vi "InStuckInIronsMode.vi"(11 "RelativeWind (0-180)":dbl) -> (3 "InStuckInIronsMode?":bool)   [LabVIEW 2012]
doc: "Checks if the boat is 1) in irons and 2) is going very slowly. There are two cutoffs - an inner angle which has lower standards for what counts as 'in irons' and a broader angle with higher standards for what counts as 'in irons'. This way if the boat is going slowly but is around, say, 25 degrees off the wind, that won't count as stuck. That same speed at 8 degrees off the wind would count as stuck.\n\nIf the boat momentum is low and the boat is in irons range this algorithm should return TRUE and we should use the sails/rudder to coax ourselves out of irons.\n\nEric Schneider, Jan. 2014"
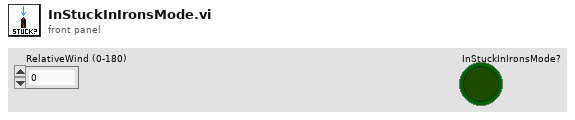
[diagram p1: front panel]
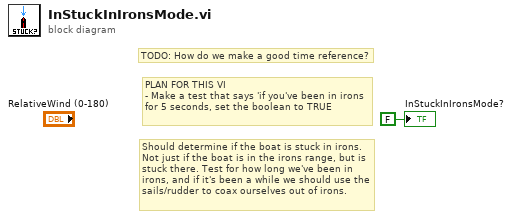
[diagram p0: block diagram]
diagram:
  # "TODO: How do we make a good time reference?"
  # "PLAN FOR THIS VI\n- Make a test that says 'if you've been in irons for 5 seconds, set the boolean to TRUE"
  # "Should determine if the boat is stuck in irons. Not just if the boat is in the irons range, but is stuck there. Test for how long we've been in irons, and if it's been a while we should use the sails/rudder to coax ourselves out of irons."
  "InStuckInIronsMode?" <- FALSE ("InStuckInIronsMode?")
